vi "CheckSubpanelDirectory.vi"(8 "error in (no error)":errorcluster, 11 "Path":path) -> (0 "error out":errorcluster, 1 "Subpanels Found?":bool, 2 "Array":path[](array[path]), 3 "Path":path)   [LabVIEW 2019, in "SMO.UI.MAUI.lvclass"]
uses:
  SMO.UI.MAUI.lvclass
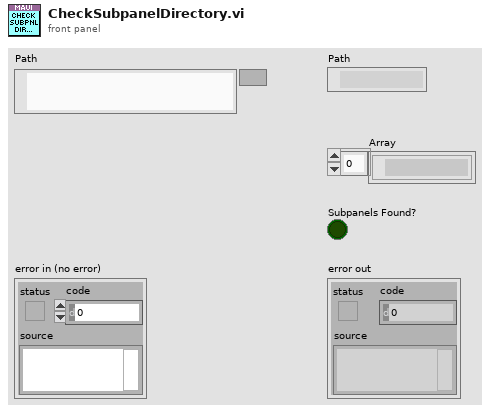
[diagram p1: front panel]
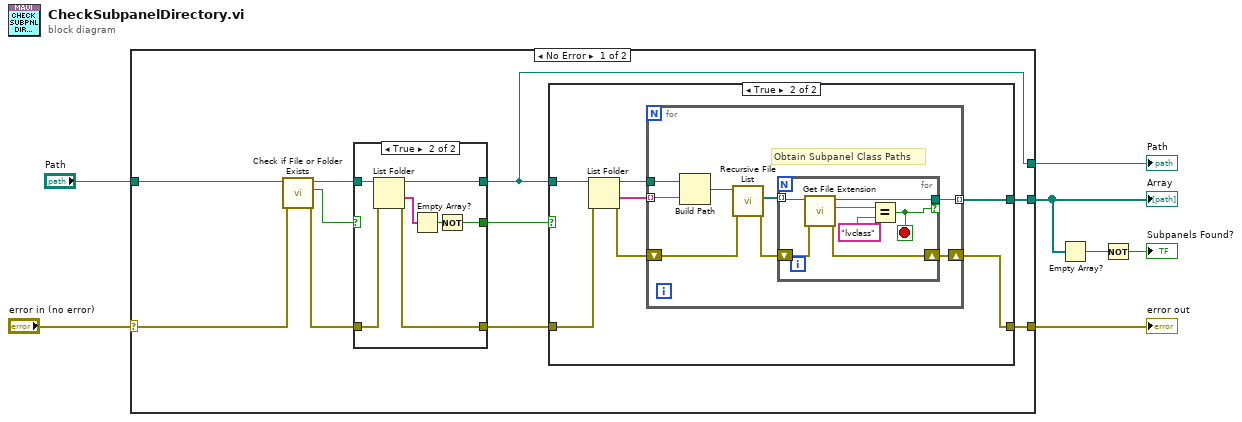
[diagram p0: block diagram]
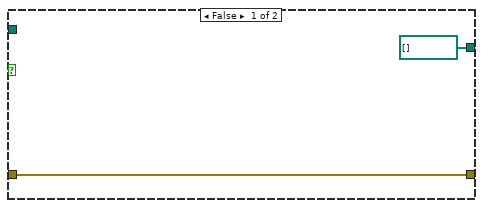
[diagram p2: hidden frame]
diagram:
  n1 = case shown="No Error" "error in (no error)" {
    selector: "error in (no error)" -> [w16 w53]
    tunnel: [w14 w53] -> w6
    tunnel: "Path" -> [w11 w52]
    tunnel: [w10 _] -> w4
    tunnel: [w8 w52] -> w3
    frame No Error {
      n2 = call <vilib>:"Check if File or Folder Exists.vi"("error in (no error)"=w16, "path"=w11) -> ("error out"=w17:errorcluster, "file or folder exists?"=w12:bool, "dup path"=w13:path)  [unwired: 7 in]
      n3 = case shown="True" w12 {
        selector: w12 -> [w43 _]
        tunnel: w13 -> [w42 w49]
        tunnel: w17 -> [w44 w51]
        tunnel: [w44 w50] -> w15
        tunnel: [w43 w47] -> w9
        tunnel: [w42 w46] -> w8
        frame False {
        }
        frame True {
          n4 = List Folder(path=w49, error in=w51) -> (path out=w46:path, folder names=w45:string[], error out=w50:errorcluster)  [unwired: 2 in, 1 out]
          n5 = Empty Array?(array=w45) -> (empty?=w48:bool)
          n6 = Not(x=w48) -> (.not. x?=w47:bool)
        }
      }
      n7 = case shown="True" w9 {
        tunnel: w8 -> [_ w23]
        tunnel: w15 -> [w19 w26]
        tunnel: [w19 w24] -> w14
        tunnel: [path[] [] w20] -> w10
        frame False {
        }
        frame True {
          n8 = List Folder(path=w23, error in=w26) -> (path out=w21:path, folder names=w22:string[], error out=w25:errorcluster)  [unwired: 2 in, 1 out]
          n9 = for {
            tunnel: w22 -> [w29] mode=indexing
            tunnel: w21 -> [w28]
            shift-right: [w33] -> w24
            shift-left: w25 -> [w32]
            tunnel: [w27] -> w20 mode=indexing
            # "Obtain Subpanel Class Paths"
            n10 = Build Path(base path=w28, name or relative path=w29) -> (appended path=w30:path)
            n11 = call <vilib>:"Recursive File List.vi"("error in (no error)"=w32, "Folder Path"=w30) -> ("error out"=w34:errorcluster, "All Files in Dir"=w31:path[])  [unwired: 5 in, 3 out]
            n12 = for {
              tunnel: w31 -> [w37] mode=indexing
              tunnel: [w36] -> w27 if=w35
              shift-right: [w40] -> w33
              shift-left: w34 -> [w41]
              stop <- w35 stop-if-true
              n13 = call <vilib>:"Get File Extension.vi"("error in (no error)"=w41, "file"=w37) -> ("error out"=w40:errorcluster, "lowercase file extension"=w39:string, "dup file"=w36:path)  [unwired: 5 in, 2 out]
              n14 = Equal?(x=w39, y="lvclass") -> (x = y?=w35:bool)
            }
          }
        }
      }
    }
    frame Error {
    }
  }
  "error out" <- w6
  "Array" <- w4
  "Path" <- w3
  n15 = Empty Array?(array=w4) -> (empty?=w2:bool)
  n16 = Not(x=w2) -> (.not. x?=→"Subpanels Found?":bool)
